vi "Image Index Operation.vi"(8 "error in (no error)":errorcluster, 10 "IndexOperation":i32, 11 "Actor in":refnum<class "Actor.lvclass">) -> (0 "error out":errorcluster, 2 "Index Out":i32, 3 "Actor out":refnum<class "Actor.lvclass">)   [LabVIEW 2015, in "Actor.lvclass"]
uses:
  Actor.lvclass
  Actor.lvclass/Actor.ctl
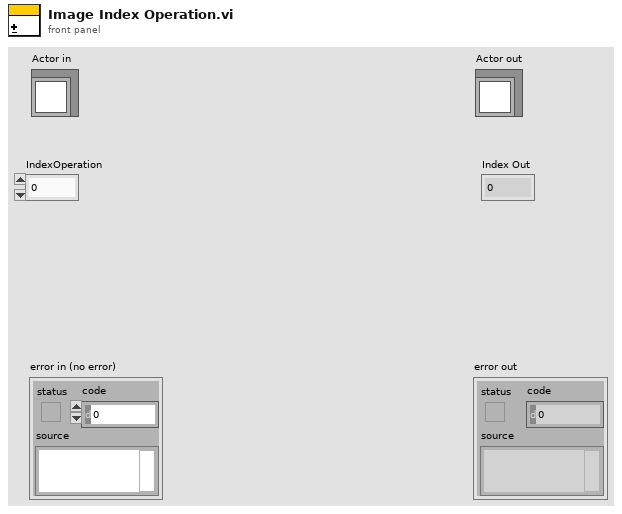
[diagram p1: front panel]
types:
  T1 = enum8{"Enabled", "Disabled", "Disabled and Grayed Out"}
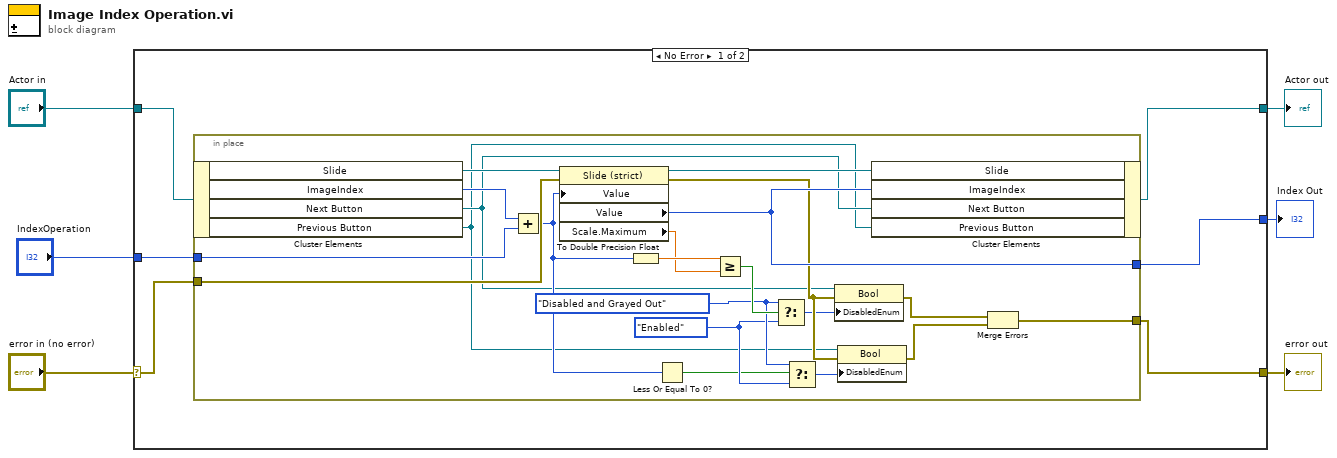
[diagram p0: block diagram]
diagram:
  n1 = case shown="No Error" "error in (no error)" {
    selector: "error in (no error)" -> [w9 w35]
    tunnel: [w8 w35] -> w5
    tunnel: [w10 w34] -> w3
    tunnel: "Actor in" -> [w12 w34]
    tunnel: "IndexOperation" -> [w11 _]
    tunnel: [w7 _] -> w1
    frame No Error {
      n2 = in-place {
        in-place-border: w11 -> [w32]
        in-place-border: w9 -> [w30]
        in-place-border: [w16] -> w8
        in-place-border: [w28] -> w7
        w21 = T1."Enabled" ("Disabled")
        w22 = T1."Disabled and Grayed Out" ("Disabled")
        n3 = in-place-cluster #1(w12) -> ("Slide"=w31:refnum<vi>, "ImageIndex"=w33:i32, "Next Button"=w15:refnum<vi>, "Previous Button"=w14:refnum<vi>)
        n4 = Add(x=w33, y=w32) -> (x+y=w20:i32)
        n5 = property class="Slide (strict)"(reference=w31, error in=w30, "Value"=w20) -> (reference out=w29:refnum<vi>, error out=w25:errorcluster, "Value"=w28:i32, "Scale.Maximum"=w13:dbl)
        n6 = To Double Precision Float(number=w20) -> (double precision float=w27:dbl)
        n7 = Less Or Equal To 0?(x=w20) -> (x <= 0?=w19:bool)
        n8 = Greater Or Equal?(x=w27, y=w13) -> (x >= y?=w26:bool)
        n9 = Select(t=w22, s=w26, f=w21) -> (s? t:f=w24:T1)
        n10 = Select(t=w22, s=w19, f=w21) -> (s? t:f=w23:T1)
        n11 = property class="Bool"(reference=w15, error in=w25, "DisabledEnum"=w24) -> (error out=w18:errorcluster)  [unwired: 1 out]
        n12 = property class="Bool"(reference=w14, error in=w25, "DisabledEnum"=w23) -> (error out=w17:errorcluster)  [unwired: 1 out]
        n13 = in-place-cluster #1("Slide"=w29, "ImageIndex"=w28, "Next Button"=w15, "Previous Button"=w14) -> (w10:refnum<class "Actor.lvclass">)
        n14 = Merge Errors(w18, w17) -> (w16:errorcluster)
      }
    }
    frame Error {
    }
  }
  "error out" <- w5
  "Actor out" <- w3
  "Index Out" <- w1
